vi "Write TEC_AO.vi"(8 "error in (no error)":errorcluster, 10 "TEC_AO":refnum<k21>, 11 "TEC Humidity Control in":refnum<class "TEC Humidity Control.lvclass">) -> (0 "error out":errorcluster, 3 "TEC Humidity Control out":refnum<class "TEC Humidity Control.lvclass">)   [LabVIEW 2016, in "TEC Humidity Control.lvclass"]
uses:
  TEC Humidity Control.lvclass
  TEC Humidity Control.lvclass/TEC Humidity Control.ctl
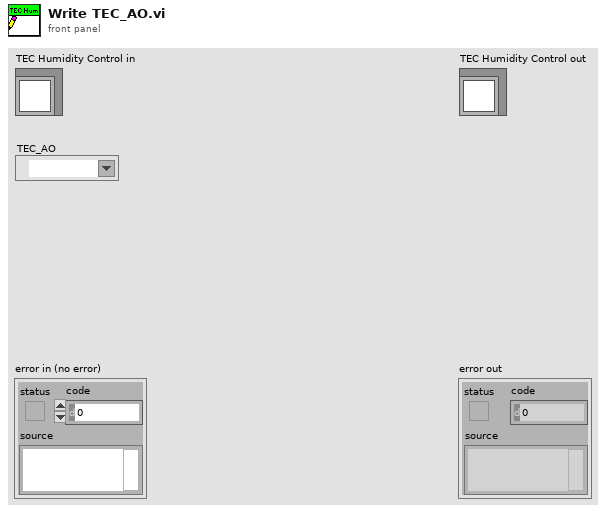
[diagram p1: front panel]
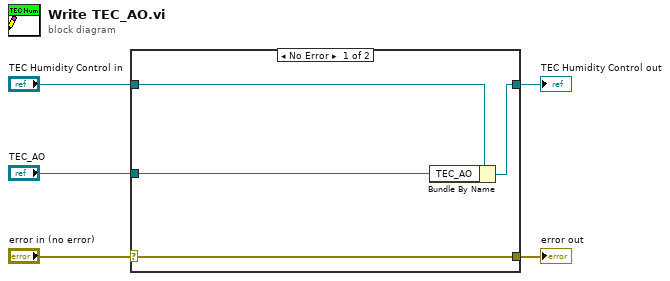
[diagram p0: block diagram]
diagram:
  n1 = case shown="No Error" "error in (no error)" {
    selector: "error in (no error)" -> [w9 w10]
    tunnel: [w9 w10] -> w4
    tunnel: [w7 w11] -> w2
    tunnel: "TEC Humidity Control in" -> [w8 w11]
    tunnel: "TEC_AO" -> [w6 _]
    frame No Error {
      n2 = Bundle By Name(cluster=w8, "TEC_AO"=w6) -> (w7:refnum<class "TEC Humidity Control.lvclass">)
    }
    frame Error {
    }
  }
  "error out" <- w4
  "TEC Humidity Control out" <- w2
